vi "Apply.vi"(8 "error in (no error)":errorcluster, 11 "DI DAQmx CFG in":refnum<class "DI DAQmx Meas Freq CFG.lvclass">) -> (0 "error out":errorcluster, 3 "DI DAQmx CFG out":refnum<class "DI DAQmx Meas Freq CFG.lvclass">)   [LabVIEW 2024, in "DI DAQmx Meas Freq CFG.lvclass"]
uses:
  DI DAQmx Meas Freq CFG.lvclass
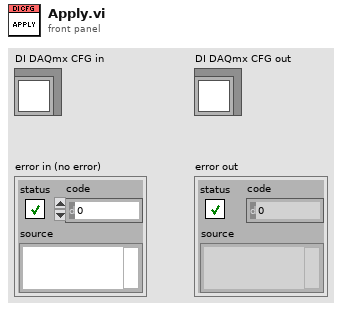
[diagram p1: front panel]
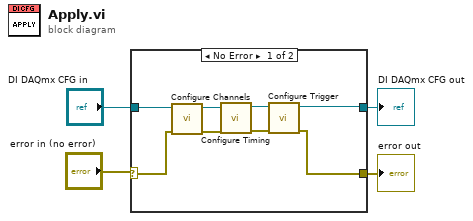
[diagram p0: block diagram]
diagram:
  n1 = case shown="No Error" "error in (no error)" {
    selector: "error in (no error)" -> [w7 w13]
    tunnel: "DI DAQmx CFG in" -> [w8 w14]
    tunnel: [w5 w14] -> w3
    tunnel: [w6 w13] -> w1
    frame No Error {
      n2 = call-dynamic "Configure Channels.vi"("error in (no error)"=w7, "DI DAQmx CFG in"=w8) -> ("error out"=w11:errorcluster, "DI DAQmx CFG out"=w12:refnum<class "DI DAQmx Meas Freq CFG.lvclass">)  [unwired: 8 in]
      n3 = call-dynamic "Configure Timing.vi"("error in"=w11, "DAQmx Base CFG in"=w12) -> ("error out"=w9:errorcluster, "DAQmx Base CFG out"=w10:refnum<class "DI DAQmx Meas Freq CFG.lvclass">)  [unwired: 8 in]
      n4 = call-dynamic "Configure Trigger.vi"("error in"=w9, "DAQmx Base CFG in"=w10) -> ("error out"=w6:errorcluster, "DAQmx Base CFG out"=w5:refnum<class "DI DAQmx Meas Freq CFG.lvclass">)  [unwired: 8 in]
    }
    frame Error {
    }
  }
  "error out" <- w1
  "DI DAQmx CFG out" <- w3
